vi "main.vi"() -> ()   [LabVIEW 2015]
uses:
  SYS/Master Controller_llb/Master Controller.lvclass
panel:
  out "String":string="Initializing..."
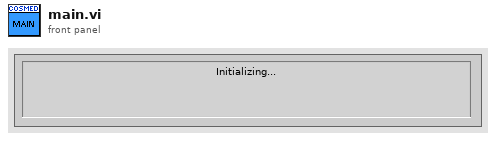
[diagram p1: front panel]
types:
  T1 = enum32{"Invalid", "Standard", "Closed", "Hidden", "Minimized", "Maximized"}
  T2 = enum32{"invalid app kind", "Development System", "Run Time System", "Student Edition", "Embedded LabVIEW", "Evaluation", "Custom"}
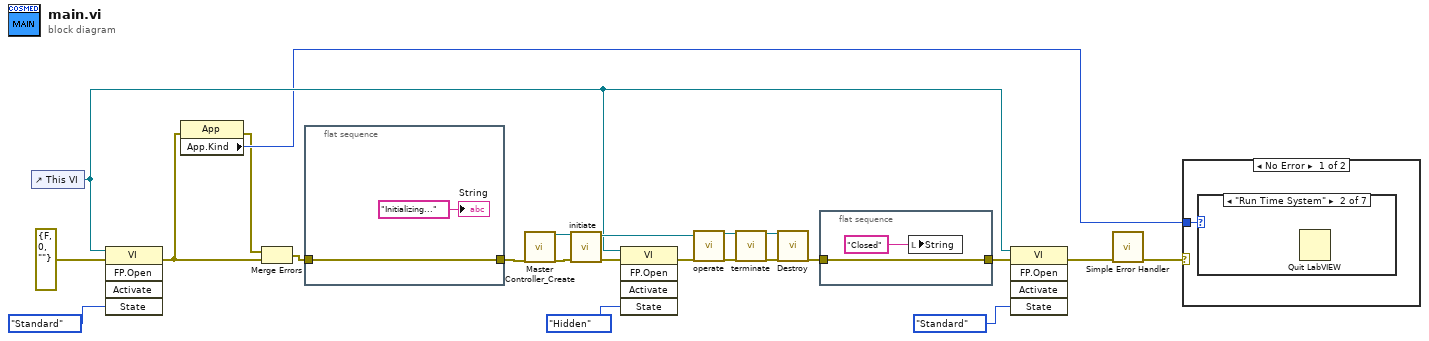
[diagram p0: block diagram]
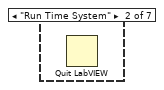
[diagram p10: hidden frame]
diagram:
  n1 = control-ref of="This VI"() -> (w15:refnum<vi>)
  n2 = invoke class="VI" method="FP.Open"(reference=w15, error in=errorcluster {"status"=FALSE, "code"=0, "source"=""} ("error in (no error)"), "State"=T1."Standard") -> (error out=w2:errorcluster)  [unwired: 2 in, 4 out]
  n3 = property class="App"(error in=w2) -> (error out=w3:errorcluster, "App.Kind"=w9:T2)  [unwired: 1 in, 1 out]
  n4 = Merge Errors(w3, w2) -> (w1:errorcluster)
  n5 = flat-sequence {
    tunnel: w1 -> [w25]
    tunnel: [w25] -> w18
    frame #0 {
      "String" <- "Initializing..." ("String")
    }
  }
  n6 = call "Master Controller_Create.vi"("error in (no error)"=w18) -> ("reference out"=w6:refnum<class "Master Controller.lvclass">, "error out"=w7:errorcluster)  [unwired: 17 in]
  n7 = call "initiate.vi"("error in (no error)"=w7, "reference in"=w6) -> ("error out"=w17:errorcluster, "reference out"=w23:refnum<class "Master Controller.lvclass">)  [unwired: 8 in]
  n8 = invoke class="VI" method="FP.Open"(reference=w15, error in=w17, "State"=T1."Hidden") -> (error out=w16:errorcluster)  [unwired: 2 in, 4 out]
  n9 = call "operate.vi"("reference in"=w23, "error in (no error)"=w16) -> ("reference out"=w22:refnum<class "Master Controller.lvclass">, "error out"=w21:errorcluster)  [unwired: 16 in]
  n10 = call "terminate.vi"("reference in"=w22, "error in (no error)"=w21) -> ("reference out"=w19:refnum<class "Master Controller.lvclass">, "error out"=w20:errorcluster)  [unwired: 16 in]
  n11 = call-dynamic "Destroy.vi"("reference in"=w19, "error in (no error)"=w20) -> ("error out"=w11:errorcluster)  [unwired: 16 in, 1 out]
  n12 = flat-sequence {
    tunnel: w11 -> [w27]
    tunnel: [w27] -> w10
    frame #0 {
      n13 = local write "String"("Closed" ("String")) -> ()
    }
  }
  n14 = invoke class="VI" method="FP.Open"(reference=w15, error in=w10, "State"=T1."Standard") -> (error out=w5:errorcluster)  [unwired: 2 in, 4 out]
  n15 = call <vilib>:"Simple Error Handler.vi"("error in (no error)"=w5) -> ("error out"=w8:errorcluster)  [unwired: 4 in, 4 out]
  n16 = case shown="No Error" w8 {
    tunnel: w9 -> [w28 w29]
    frame No Error {
      n17 = case shown="\"Run Time System\"" w28 {
        frame "invalid app kind", Default {
        }
        frame "Run Time System" {
          n18 = Quit LabVIEW() -> ()  [unwired: 1 in]
        }
        frame "Student Edition" {
        }
        frame "Embedded LabVIEW" {
        }
        frame "Evaluation" {
        }
        frame "Custom" {
        }
        frame "Development System" {
        }
      }
    }
    frame Error {
      n19 = case shown="\"Development System\"" w29 {
        frame "invalid app kind", Default {
        }
        frame "Run Time System" {
          n20 = Quit LabVIEW() -> ()  [unwired: 1 in]
        }
        frame "Student Edition" {
        }
        frame "Embedded LabVIEW" {
        }
        frame "Evaluation" {
        }
        frame "Custom" {
        }
        frame "Development System" {
        }
      }
    }
  }
